vi "readAI.vi"(7 "address":string, 8 "error in (no error)":errorcluster) -> (0 "error out":errorcluster, 2 "input signal":waveform(dbl)[](array[waveform]))   [LabVIEW 2016]
doc: "API to get the AI waveforms.\n\nIf address=\"\", this API reads from localhost\nIf address is remote lockin, you need to add this computer to allowed whitelist on the lockin computer you are trying to access."
uses:
  RemoteControl/Typedefs/Remote-SMO-Commands-Enum.ctl
  RemoteControl/Typedefs/PrivateEvents--LockinRemoteControl.setAI.ctl
  RemoteControl/LockinRemoteControl.lvclass
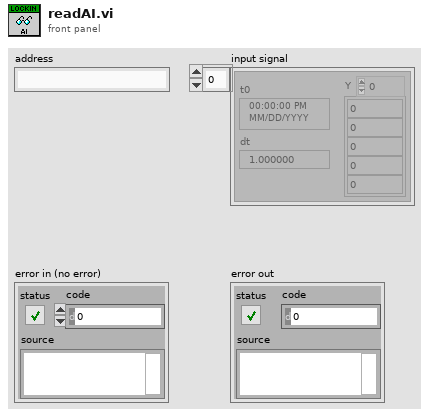
[diagram p1: front panel]
types:
  T1 = typedef "LockinRemoteControl.lvclass/PrivateEvents--LockinRemoteControl.setAI.ctl" = waveform(dbl)[]
  T2 = typedef "LockinRemoteControl.lvclass/Remote-SMO-Commands-Enum.ctl" = enum16{"configAO", "configREF", "configREFfilter", "configIVmode", "configRemote", "configReset", "configSampling", "assertTrigger", "getAO", "getAI", "getResults", "getTrigger", "getIVmode", "getSampling", "getAOconfig", "getREFconfig", "getREFfilter", "ACK", "UNK", "CLOSE", "configGain", "getGain"}
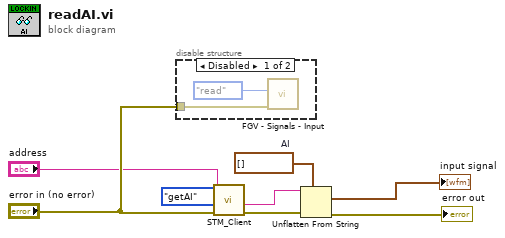
[diagram p0: block diagram]
diagram:
  w7 = T1 []  # AI
  n1 = disable-structure shown="Disabled" {
    disable-tunnel: "error in (no error)" -> [w9 _]
    frame Disabled {
      n2 = call "FGV - Signals - Input.vi"("error in"=w9, "Function"=enum16{"write", "read"}."read") -> ()  [unwired: 4 in, 2 out]
    }
    frame Enabled {
    }
  }
  n3 = call "STM_Client.vi"("error in (no error)"="error in (no error)", "Command"=Remote-SMO-Commands-Enum."getAI", "address"="address") -> ("error out"=w5:errorcluster, "data received from server"=w4:string)  [unwired: 7 in]
  n4 = Unflatten From String(type=w7, binary string=w4, error in (no error)=w5) -> (value=→"input signal":T1, error out=→"error out":errorcluster)  [unwired: 2 in, 1 out]
